vi "Read RingdownConfig.vi"(8 "error in (no error)":errorcluster, 11 "RingdownPlugin in":refnum<class "RingdownPlugin.lvclass">) -> (0 "error out":errorcluster, 2 "RingdownConfig":T1={"Config"={"Addmod"=-1, "Scalmod"=0, "Lpocon"=-1, "Pircon"=-1, "Dmodes"=0, "Lpmcon"=3, "Lpacon"=1, "Fbcon"=1, "Ordcon"=1, "Trimre"=-1.0, "Ftrimh"=-1.0, "Ftriml"=-1.0}, "Window"={"StOffset"=1, "EndOffset"=100, "Length"=10000}, "V index"=0, "I index"=3, "PosSeq"=FALSE} {"Config"."Fbcon" items=["", "Forward", "Forward-Backward", "Backward"]; "Config"."Lpmcon" items=["", "Correlation", "Pre-windowed", "Covariance", "Post-windowed"]; "Config"."Lpacon" items=["", "SVD with possible rank reduction", "QR reduction via LAPACK", "Total least squares via SVD"]}, 3 "RingdownPlugin out":refnum<class "RingdownPlugin.lvclass">)   [LabVIEW 2017, in "AppPlugins.lvlib" / "RingdownPlugin.lvclass"]
uses:
  RingdownPlugin.lvclass
  PublicAPI/TypeDef/RingdownConfig.ctl
  RingdownPlugin.lvclass/RingdownPlugin.ctl
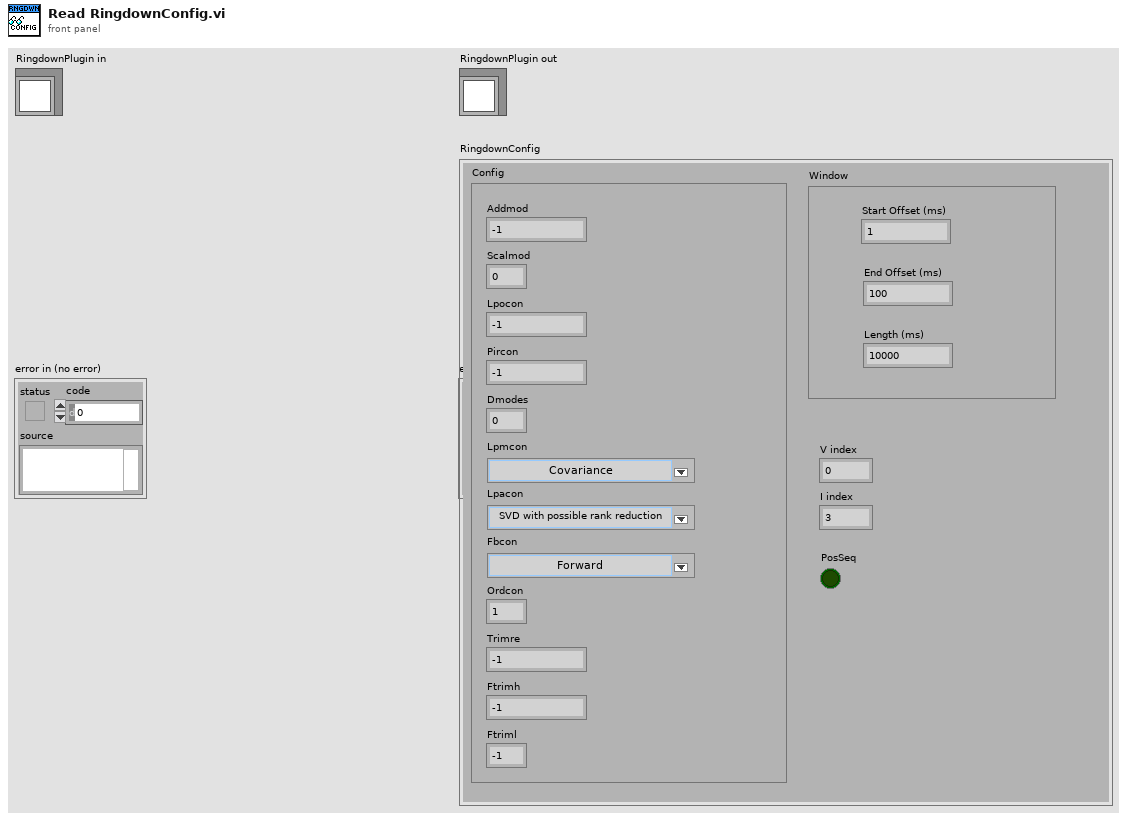
[diagram p1: front panel]
types:
  T1 = typedef "AppPlugins.lvlib/RingdownPlugin.lvclass/RingdownConfig.ctl" = cluster{"Config":cluster{"Addmod":i32, "Scalmod":i32, "Lpocon":i32, "Pircon":i32, "Dmodes":i32, "Lpmcon":u16, "Lpacon":u16, "Fbcon":u16, "Ordcon":i32, "Trimre":dbl, "Ftrimh":dbl, "Ftriml":dbl}, "Window":cluster{"StOffset":i32, "EndOffset":i32, "Length":i32}, "V index":i32, "I index":i32, "PosSeq":bool}
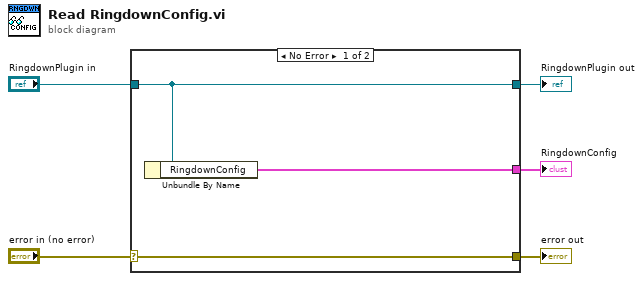
[diagram p0: block diagram]
diagram:
  n1 = case shown="No Error" "error in (no error)" {
    selector: "error in (no error)" -> [w8 w9]
    tunnel: [w8 w9] -> w4
    tunnel: [w7 w10] -> w2
    tunnel: "RingdownPlugin in" -> [w7 w10]
    tunnel: [w6 _] -> w1
    frame No Error {
      n2 = Unbundle By Name(w7) -> ("RingdownConfig"=w6:T1)
    }
    frame Error {
    }
  }
  "error out" <- w4
  "RingdownPlugin out" <- w2
  "RingdownConfig" <- w1
